vi "PathPlanner_PointTowardsZone_New.vi"(7 "Name":string, 8 "MaxPosition":dbl, 9 "MinPosition":dbl, 10 "RotationOffset":T1={"VALUE"=0.0, "COS"=1.0, "SIN"=0.0} {"SIN" format="%13.4f"; "COS" format="%13.4f"; "VALUE" format="%13.4f"}, 11 "TargetPosition":T2 {"Y" format="%14.3f"; "X" format="%14.3f"}) -> (3 "PointTowardsZone":T3={"RotationOffset"={"VALUE"=0.0, "COS"=1.0, "SIN"=0.0}, "Name"="", "TargetPosition"={"X"=0.0, "Y"=0.0}, "MinPosition"=0.0, "MaxPosition"=0.0} {"TargetPosition"."Y" format="%14.3f"; "TargetPosition"."X" format="%14.3f"; "RotationOffset"."SIN" format="%13.4f"; "RotationOffset"."COS" format="%13.4f"; "RotationOffset"."VALUE" format="%13.4f"})   [LabVIEW 2019, in "PathPlanner24.lvlib"]
doc: "Create a new cluster containing zone on a path that will force the robot to point towards a position on the field\n\nInputs:\n - name - string - The name of this zone. Used for point towards zone triggers\n - targetPosition - translation2d - The target field position in meters\n - rotationOffset - rotation2d - A rotation offset to add on top of the angle to the target position. For example, if you want the robot to point away from the target position, use a rotation offset of 180 degrees. (Default: 0.0)\n - minPosition - double - Starting waypoint relative position of the zone\n - maxPosition - double - End waypoint relative position of the zone\n\nOutputs:\n - PointTowardsZone - cluster - defined point towards zone data structure"
uses:
  PathPlanner24.lvlib
  TypeDef/PathPlannerPointTowardsZone.ctl
  <vilib>/Rock Robotics/WPI/ThirdParty/JAS_Junk/TrajLib/TypeDef/ROTATION2D.ctl
  <vilib>/Rock Robotics/WPI/ThirdParty/JAS_Junk/TrajLib/TypeDef/TRANSLATION2D.ctl
  <vilib>/Rock Robotics/WPI/ThirdParty/JAS_Junk/TrajLib/Trajectory_Library.lvlib
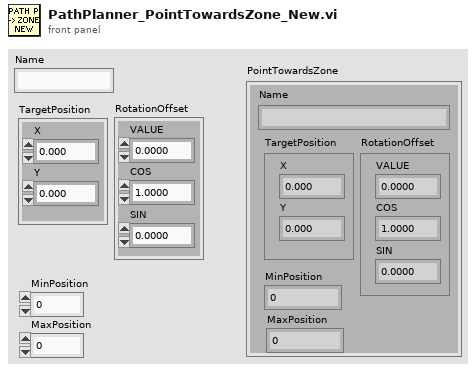
[diagram p1: front panel]
types:
  T1 = typedef "Trajectory_Library.lvlib/ROTATION2D.ctl" = cluster{"VALUE":dbl, "COS":dbl, "SIN":dbl}
  T2 = typedef "Trajectory_Library.lvlib/TRANSLATION2D.ctl" = cluster{"X":dbl, "Y":dbl}
  T3 = typedef "PathPlanner24.lvlib/PathPlannerPointTowardsZone.ctl" = cluster{"RotationOffset":T1, "Name":string, "TargetPosition":T2, "MinPosition":dbl, "MaxPosition":dbl}
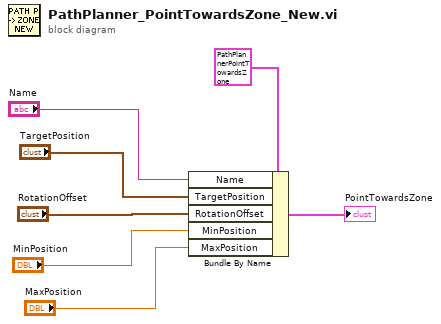
[diagram p0: block diagram]
diagram:
  n1 = Bundle By Name(cluster=T3 {"RotationOffset"={"VALUE"=0.0, "COS"=1.0, "SIN"=0.0}, "Name"="", "TargetPosition"={"X"=0.0, "Y"=0.0}, "MinPosition"=0.0, "MaxPosition"=0.0} ("PointTowardsZone"), "Name"="Name", "TargetPosition"="TargetPosition", "RotationOffset"="RotationOffset", "MinPosition"="MinPosition", "MaxPosition"="MaxPosition") -> (→"PointTowardsZone":T3)
